vi "gen_string_message_missing_calibration_valves.vi"(0 "Missing Calibration Refs":T1) -> (7 "String":string)   [LabVIEW 2016]
panel:
  in  "Missing Valves":u16[](array[ring]) items=["A1", "A2", "A3", "A4", "B1", "B2", "B3", "B4", "B5", "B6", "B7", "B8", "A5"]
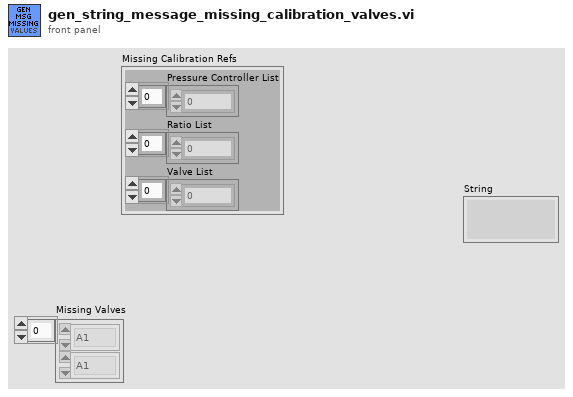
[diagram p1: front panel]
types:
  T1 = cluster{"Pressure Controller List":u8[], "Ratio List":dbl[], "Valve List":u16[]}
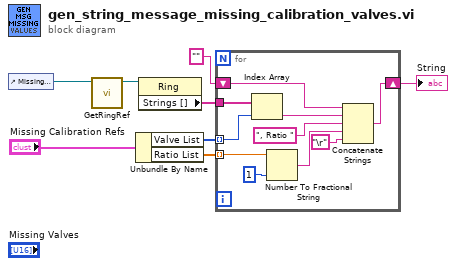
[diagram p0: block diagram]
diagram:
  n1 = control-ref of="Missing Valves"() -> (w8:refnum<vi>)
  n2 = call "GetRingRef.vi"("Array Reference"=w8) -> ("Ring Reference"=w4:refnum<vi>)  [unwired: 9 in, 1 out]
  n3 = Unbundle By Name("Missing Calibration Refs") -> ("Valve List"=w2:u16[], "Ratio List"=w1:dbl[])
  n4 = property class="Ring"(reference=w4) -> ("Strings []"=w7:string[])  [unwired: 1 in, 2 out]
  n5 = for {
    tunnel: w2 -> [w17] mode=indexing
    tunnel: w7 -> [w18]
    tunnel: w1 -> [w16] mode=indexing
    shift-right: [w12] -> w5
    shift-left: "" -> [w10]
    n6 = Index Array(array=w18, index=w17) -> (element=w15:string)
    n7 = Number To Fractional String(number=w16, precision (6)=i16 1) -> (F-format string=w13:string)  [unwired: 2 in]
    n8 = Concatenate Strings(w10, w15, ", Ratio " ("string"), w13, "\r") -> (w12:string)
  }
  "String" <- w5
